vi "Model - Set RT data.vi"(8 "error in (no error)":errorcluster, 10 "RT data":dbl[][](array[numeric]), 11 "View Model":T1) -> (0 "error out":errorcluster, 3 "View Model":T1)   [LabVIEW 2017]
doc: "Set actual value of RT data into DVR"
uses:
  Controls/View Model.ctl
  Controls/Shared Model.ctl
  Error Handler/Controls/Error Model.ctl
  Error Handler/Controls/Error Event.ctl
  Error Handler/Controls/Error Type.ctl
  Controller/Controls/Controller Model.ctl
  Controller/Controls/Controller Event.ctl
  Controller/Controls/Controller Command.ctl
  Controller/Controls/Controller Overhead.ctl
  Real-Time/RT Status.ctl
  Real-Time/RT Loop Status.ctl
  Controller/Controls/Controller NStream.ctl
  Controller/Controls/Controller DAQ Data.ctl
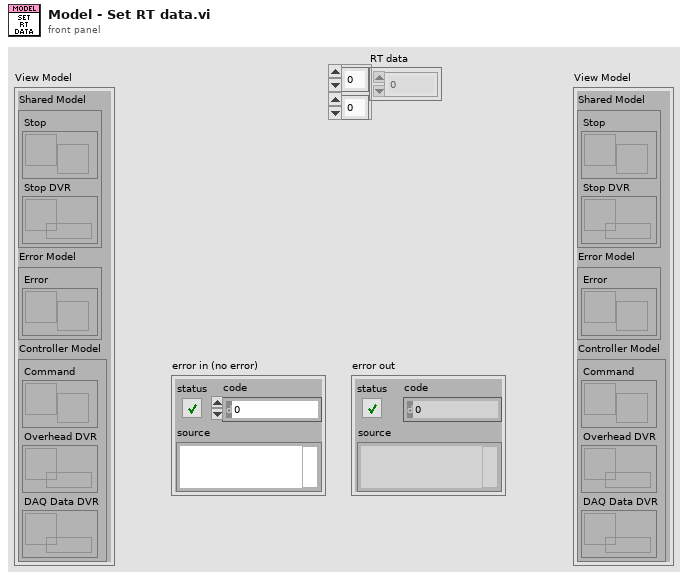
[diagram p1: front panel]
types:
  T1 = typedef "View Model.ctl" = cluster{"Shared Model":T2, "Error Model":T3, "Controller Model":T4}
  T2 = typedef "Shared Model.ctl" = cluster{"Stop":refnum<user-event>, "Stop DVR":refnum<data-value>}
  T3 = typedef "Error Model.ctl" = cluster{"Error":refnum<user-event>}
  T4 = typedef "Controller Model.ctl" = cluster{"Command":refnum<user-event>, "Overhead DVR":refnum<data-value>, "DAQ Data DVR":refnum<data-value>}
  T5 = typedef "Controller Overhead.ctl" = cluster{"Start":bool, "Numeric":dbl, "Blink CNTRLR1":bool, "Blink CNTRLR2":bool, "RT Status":T6, "NStream2":refnum<k21>, "RT data":dbl[][], "NStream":T8}
  T6 = typedef "RT Status.ctl" = cluster{"Status TCL1":T7, "Status TCL2":T7, "Status NPL":T7, "Connected?":bool}
  T7 = typedef "RT Loop Status.ctl" = cluster{"Duration, us":dbl, "Late Counter":i32, "Timeout, us":u32}
  T8 = typedef "Controller NStream.ctl" = cluster{"Endpoint":refnum<k21>, "exist?":bool}
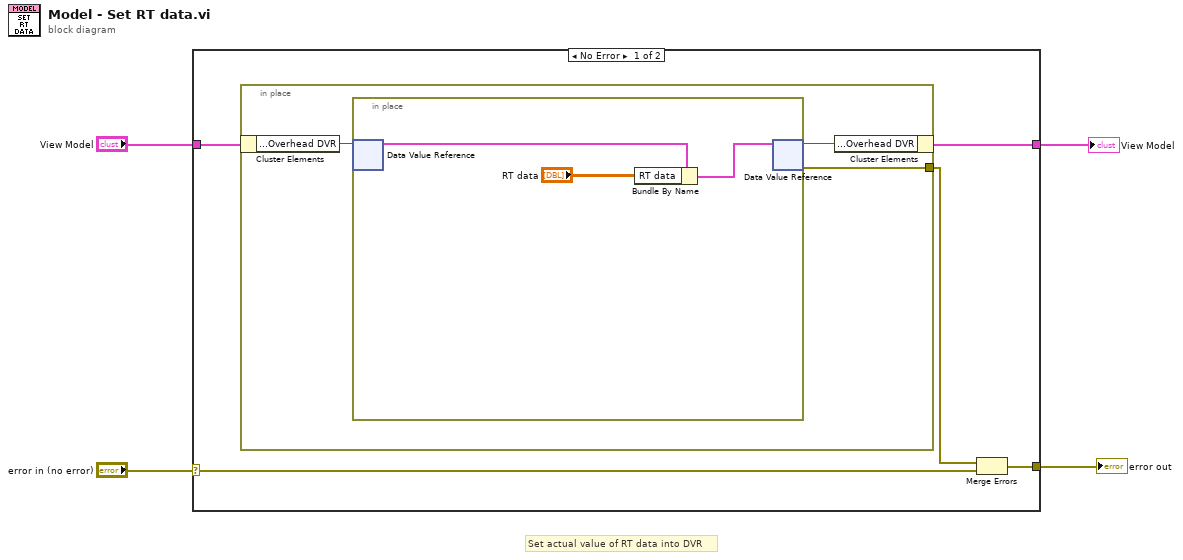
[diagram p0: block diagram]
diagram:
  # "Set actual value of RT data into DVR"
  n1 = case shown="No Error" "error in (no error)" {
    selector: "error in (no error)" -> [w6 w16]
    tunnel: "View Model" -> [w9 w17]
    tunnel: [w8 w17] -> w2
    tunnel: [w5 w16] -> w1
    frame No Error {
      n2 = in-place {
        in-place-border: [w10] -> w7
        n3 = in-place-cluster #1(w9) -> ("Controller Model.Overhead DVR"=w12:refnum<data-value>)
        n4 = in-place {
          n5 = in-place-dvr #2(w12) -> (w15:T5)  [unwired: 1 out]
          n6 = Bundle By Name(cluster=w15, "RT data"="RT data") -> (w14:T5)
          n7 = in-place-dvr #2(w14) -> (w11:refnum<data-value>, w10:errorcluster)
        }
        n8 = in-place-cluster #1("Controller Model.Overhead DVR"=w11) -> (w8:T1)
      }
      n9 = Merge Errors(w7, w6) -> (w5:errorcluster)
    }
    frame Error {
    }
  }
  "View Model" <- w2
  "error out" <- w1
